vi "Top Box Json Reply Parser.vi"(11 "value":T5 {"DomeStatus"."LowerDoorEl" format="%.2f"; "DomeStatus"."UpperDoorEl" format="%.2f"}) -> (3 "output cluster":T4 {"DomeStatus"."LowerDoorEl" format="%.2f"; "DomeStatus"."UpperDoorEl" format="%.2f"})   [LabVIEW 2019]
uses:
  RT Controls/TopBox Reply.ctl
  RT Controls/Top Dome Control.ctl
  RT Controls/Top Dome Status String.ctl
  RT Controls/TopBox Config.ctl
  RT Controls/Top Dome Status.ctl
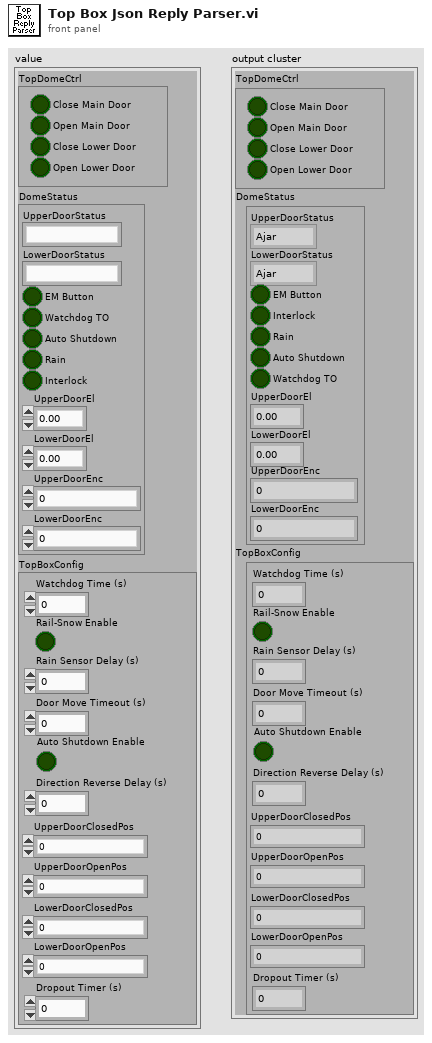
[diagram p1: front panel]
types:
  T1 = typedef "Top Dome Control.ctl" = cluster{"OpenLowerDoor":bool, "CloseLowerDoor":bool, "OpenMainDoor":bool, "CloseMainDoor":bool}
  T2 = typedef "Top Dome Status.ctl" = cluster{"UpperDoorStatus":enum16{"Ajar", "Open", "Shut", "Error"}, "LowerDoorStatus":enum16{"Ajar", "Shut", "Open", "Error"}, "EM Button":bool, "WDTime":bool, "AutoShut":bool, "Rain":bool, "Interlock":bool, "UpperDoorEl":dbl, "LowerDoorEl":dbl, "UpperDoorEnc":u64, "LowerDoorEnc":u64}
  T3 = typedef "TopBox Config.ctl" = cluster{"WatchdogTim":i32, "RainEn":bool, "DoorMoveTO":i32, "AutoShutEn":bool, "DirRevDel":i32, "UpperClosedEnc":u64, "UpperOpenEnc":u64, "LowerClosedEnc":u64, "LowerOpenEnc":u64, "RainTim":i32, "DropoutTim":i32}
  T4 = cluster{"TopDomeCtrl":T1, "DomeStatus":T2, "TopBoxConfig":T3}
  T5 = typedef "TopBox Reply.ctl" = cluster{"TopDomeCtrl":T1, "DomeStatus":T6, "TopBoxConfig":T3}
  T6 = typedef "Top Dome Status String.ctl" = cluster{"UpperDoorStatus":string, "LowerDoorStatus":string, "EM Button":bool, "WDTime":bool, "AutoShut":bool, "Rain":bool, "Interlock":bool, "UpperDoorEl":dbl, "LowerDoorEl":dbl, "UpperDoorEnc":u64, "LowerDoorEnc":u64}
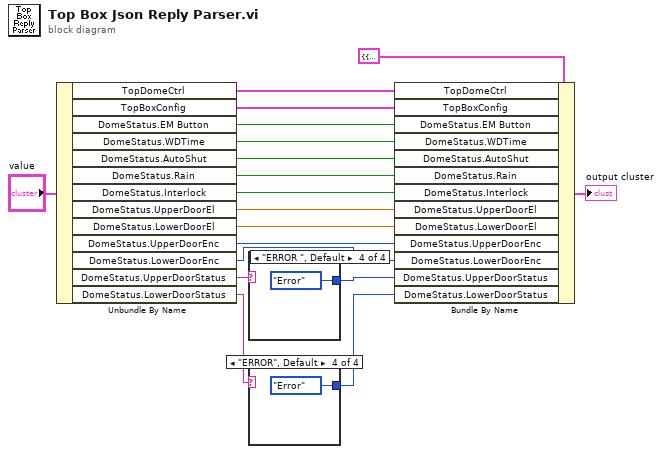
[diagram p0: block diagram]
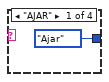
[diagram p2: hidden frame]
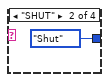
[diagram p3: hidden frame]
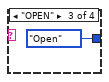
[diagram p4: hidden frame]
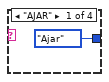
[diagram p5: hidden frame]
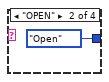
[diagram p6: hidden frame]
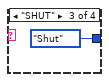
[diagram p7: hidden frame]
diagram:
  n1 = Unbundle By Name("value") -> ("TopDomeCtrl"=w3:T1, "TopBoxConfig"=w4:T3, "DomeStatus.EM Button"=w5:bool, "DomeStatus.WDTime"=w6:bool, "DomeStatus.AutoShut"=w7:bool, "DomeStatus.Rain"=w8:bool, "DomeStatus.Interlock"=w9:bool, "DomeStatus.UpperDoorEl"=w10:dbl, "DomeStatus.LowerDoorEl"=w11:dbl, "DomeStatus.UpperDoorEnc"=w12:u64, "DomeStatus.LowerDoorEnc"=w13:u64, "DomeStatus.UpperDoorStatus"=w14:string, "DomeStatus.LowerDoorStatus"=w17:string)
  n2 = case shown="\"ERROR \", Default" w14 {
    tunnel: [enum16{"Ajar", "Open", "Shut", "Error"}."Ajar" ("DomeStatus.UpperDoorStatus") enum16{"Ajar", "Open", "Shut", "Error"}."Open" ("DomeStatus.UpperDoorStatus") enum16{"Ajar", "Open", "Shut", "Error"}."Shut" ("DomeStatus.UpperDoorStatus") enum16{"Ajar", "Open", "Shut", "Error"}."Error" ("DomeStatus.UpperDoorStatus")] -> w15
    frame "AJAR" {
    }
    frame "OPEN" {
    }
    frame "SHUT" {
    }
    frame "ERROR ", Default {
    }
  }
  n3 = case shown="\"ERROR\", Default" w17 {
    tunnel: [enum16{"Ajar", "Shut", "Open", "Error"}."Ajar" ("DomeStatus.LowerDoorStatus") enum16{"Ajar", "Shut", "Open", "Error"}."Shut" ("DomeStatus.LowerDoorStatus") enum16{"Ajar", "Shut", "Open", "Error"}."Open" ("DomeStatus.LowerDoorStatus") enum16{"Ajar", "Shut", "Open", "Error"}."Error" ("DomeStatus.LowerDoorStatus")] -> w16
    frame "AJAR" {
    }
    frame "SHUT" {
    }
    frame "OPEN" {
    }
    frame "ERROR", Default {
    }
  }
  n4 = Bundle By Name(cluster=T4 {"TopDomeCtrl"={"OpenLowerDoor"=FALSE, "CloseLowerDoor"=FALSE, "OpenMainDoor"=FALSE, "CloseMainDoor"=FALSE}, "DomeStatus"={"UpperDoorStatus"=enum."Ajar", "LowerDoorStatus"=enum."Ajar", "EM Button"=FALSE, "WDTime"=FALSE, "AutoShut"=FALSE, "Rain"=FALSE, "Interlock"=FALSE, "UpperDoorEl"=0.0, "LowerDoorEl"=0.0, "UpperDoorEnc"=0, "LowerDoorEnc"=0}, "TopBoxConfig"={"WatchdogTim"=0, "RainEn"=FALSE, "DoorMoveTO"=0, "AutoShutEn"=FALSE, "DirRevDel"=0, "UpperClosedEnc"=0, "UpperOpenEnc"=0, "LowerClosedEnc"=0, "LowerOpenEnc"=0, "RainTim"=0, "DropoutTim"=0}} ("output cluster"), "TopDomeCtrl"=w3, "TopBoxConfig"=w4, "DomeStatus.EM Button"=w5, "DomeStatus.WDTime"=w6, "DomeStatus.AutoShut"=w7, "DomeStatus.Rain"=w8, "DomeStatus.Interlock"=w9, "DomeStatus.UpperDoorEl"=w10, "DomeStatus.LowerDoorEl"=w11, "DomeStatus.UpperDoorEnc"=w12, "DomeStatus.LowerDoorEnc"=w13, "DomeStatus.UpperDoorStatus"=w15, "DomeStatus.LowerDoorStatus"=w16) -> (→"output cluster":T4)
